vi "Lookup Implementation.vi"(8 "error in (no error)":errorcluster, 10 "Implementation Tag":string, 11 "Polymorphic VI Type in":refnum<class "Polymorphic VI Type.lvclass">) -> (0 "error out":errorcluster, 2 "Found?":bool, 3 "Polymorphic VI Type out":refnum<class "Polymorphic VI Type.lvclass">)   [LabVIEW 2020, in "Peek Window.lvlib" / "Polymorphic VI Type.lvclass"]
uses:
  Polymorphic VI Type.lvclass
  D:/Code/VI-Peek/source/Peek Window/VI Types/Standard VI Type/Standard VI Type.lvclass
  Polymorphic VI Type.lvclass/Polymorphic VI Type.ctl
  Selected Item Enum.ctl
  Standard VI Type/Standard VI Type.lvclass/Standard VI Type.ctl
  Standard VI Type/Read VI Refnum.vi
  Standard VI Type/Read Full Qualified Name.vi
  Standard VI Type/Write VI Refnum.vi
  Standard VI Type/Write Full Qualified Name.vi
  Implementation VI Type/Implementation VI Type.lvclass
  <vilib>/Utility/error.llb/Error Cluster From Error Code.vi
  <vilib>/ErrorRing/Error Ring.xnode
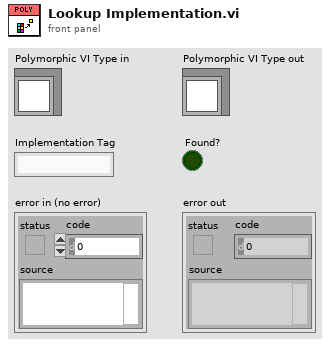
[diagram p1: front panel]
types:
  T1 = typedef "Peek Window.lvlib/Polymorphic VI Type.lvclass/Selected Item Enum.ctl" = enum16{"Polymorphic", "Instance"}
  T2 = cluster{"VIPath":path, "Menu Name":string, "Selector Name":string}[]
  T3 = map{string, refnum<class "Implementation VI Type.lvclass">}
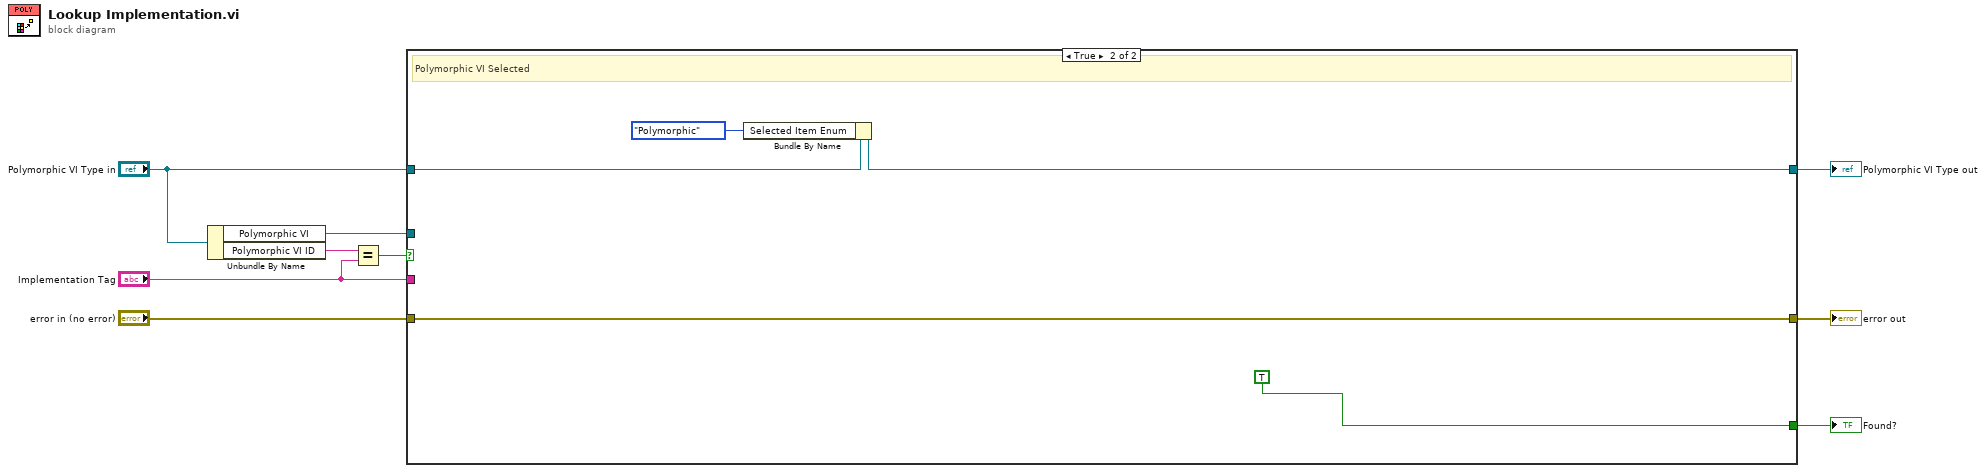
[diagram p0: block diagram]
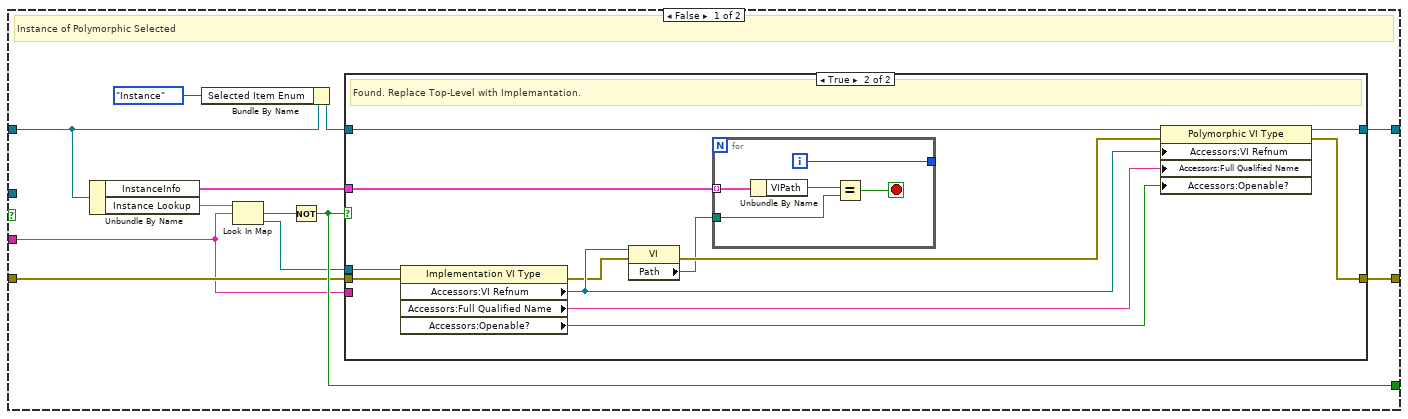
[diagram p2: hidden frame]
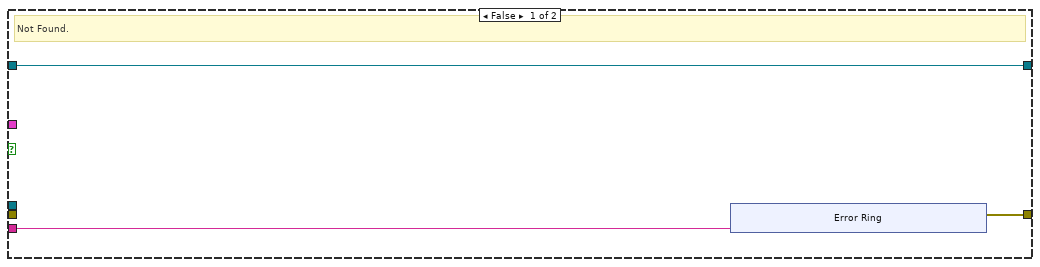
[diagram p3: hidden frame]
diagram:
  n1 = Unbundle By Name("Polymorphic VI Type in") -> ("Polymorphic VI"=w1:refnum<class "Standard VI Type.lvclass">, "Polymorphic VI ID"=w2:string)
  n2 = Equal?(x=w2, y="Implementation Tag") -> (x = y?=w4:bool)
  n3 = case shown="True" w4 {
    tunnel: [w20 w50] -> w9
    tunnel: [w18 TRUE] -> w8
    tunnel: [w17 w52] -> w7
    tunnel: "Polymorphic VI Type in" -> [w12 w49]
    tunnel: "Implementation Tag" -> [w14 _]
    tunnel: w1 -> [_ _]
    tunnel: "error in (no error)" -> [w15 w52]
    frame False {
      # "Instance of Polymorphic Selected"
      n4 = Unbundle By Name(w12) -> ("InstanceInfo"=w10:T2, "Instance Lookup"=w21:T3)
      n5 = Bundle By Name(cluster=w12, "Selected Item Enum"=Selected_Item_Enum."Instance") -> (w13:refnum<class "Polymorphic VI Type.lvclass">)
      n6 = Look In Map(map=w21, key=w14) -> (key not found?=w19:bool, value=w16:refnum<class "Implementation VI Type.lvclass">)  [unwired: 1 in]
      n7 = Not(x=w19) -> (.not. x?=w18:bool)
      n8 = case shown="True" w18 {
        tunnel: w13 -> [w24 w33]
        tunnel: [w24 w43] -> w20
        tunnel: [w22 w42] -> w17
        tunnel: w16 -> [_ w41]
        tunnel: w15 -> [_ w40]
        tunnel: w14 -> [w23 _]
        tunnel: w10 -> [_ w35]
        frame False {
          # "Not Found."
          n9 = xnode "Error Ring"("parameter 0"=w23) -> ("error out"=w22:errorcluster)
        }
        frame True {
          # "Found. Replace Top-Level with Implemantation."
          n10 = property class="Implementation VI Type"(reference=w41, error in=w40) -> (error out=w37:errorcluster, "Accessors:VI Refnum"=w38:refnum<vi>, "Accessors:Full Qualified Name"=w39:string, "Accessors:Openable?"=w32:bool)  [unwired: 1 out]
          n11 = property class="VI"(reference=w38, error in=w37) -> (error out=w36:errorcluster, "Path"=w34:path)  [unwired: 1 out]
          n12 = for {
            tunnel: w35 -> [w48] mode=indexing
            tunnel: w34 -> [w46]
            tunnel: [w44] -> _
            i -> [w44]
            stop <- w45 stop-if-true
            n13 = Unbundle By Name(w48) -> ("VIPath"=w47:path)
            n14 = Equal?(x=w47, y=w46) -> (x = y?=w45:bool)
          }
          n15 = property class="Polymorphic VI Type"(reference=w33, error in=w36, "Accessors:VI Refnum"=w38, "Accessors:Full Qualified Name"=w39, "Accessors:Openable?"=w32) -> (reference out=w43:refnum<class "Polymorphic VI Type.lvclass">, error out=w42:errorcluster)
        }
      }
    }
    frame True {
      # "Polymorphic VI Selected"
      n16 = Bundle By Name(cluster=w49, "Selected Item Enum"=Selected_Item_Enum."Polymorphic") -> (w50:refnum<class "Polymorphic VI Type.lvclass">)
    }
  }
  "error out" <- w7
  "Polymorphic VI Type out" <- w9
  "Found?" <- w8
